vi "Get Entity Details.vi"(8 "error in (no error)":errorcluster, 10 "Entity Type":i32, 11 "Entity Table in":refnum<class "Entity Table.lvclass">) -> (0 "error out":errorcluster, 2 "Entity Details":cluster{"Name":string, "Status":string}[](array[cluster]), 3 "Entity Table out":refnum<class "Entity Table.lvclass">)   [LabVIEW 2020, in "Entity Table.lvclass"]
doc: "Copy out the details of one set of Entities. This is intended to aid in creating a status display."
uses:
  Entity Table.lvclass
  Entity Table.lvclass/Entity Table.ctl
  Entity Data.ctl
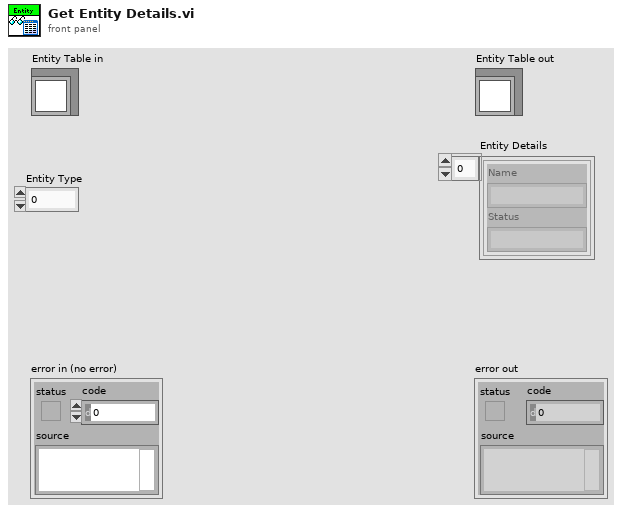
[diagram p1: front panel]
types:
  T1 = typedef "Entity Table.lvclass/Entity Data.ctl" = cluster{"Name":string, "Status":string}
  T2 = typedef "Entity Table.lvclass/Entity Table Element.ctl" = cluster{"Entity":refnum<class "Message Enqueuer.lvclass">[], "Entity Data":T1[]}
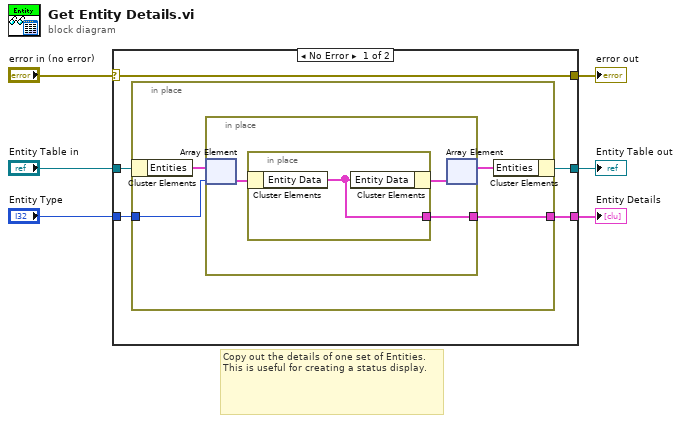
[diagram p0: block diagram]
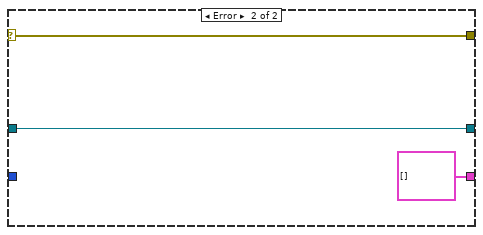
[diagram p2: hidden frame]
diagram:
  # "Copy out the details of one set of Entities.  This is useful for creating a status display."
  n1 = case shown="No Error" "error in (no error)" {
    selector: "error in (no error)" -> [w11 w22]
    tunnel: [w11 w22] -> w5
    tunnel: [w8 w21] -> w3
    tunnel: "Entity Table in" -> [w10 w21]
    tunnel: "Entity Type" -> [w9 _]
    tunnel: [w7 T1[] [] ("Entity Data")] -> w1
    frame No Error {
      n2 = in-place "In Place Element Structure" {
        in-place-border: w9 -> [w14]
        in-place-border: [w12] -> w7
        n3 = in-place-cluster #1 ("Unbundle / Bundle Elements")(w10) -> ("Entities"=w15:T2[])
        n4 = in-place "In Place Element Structure" {
          in-place-border: [w16] -> w12
          n5 = in-place-array #2 ("Array Index / Replace Elements")(w15, w14) -> (w18:T2)
          n6 = in-place "In Place Element Structure" {
            in-place-border: [w19] -> w16
            n7 = in-place-cluster #3 ("Unbundle / Bundle Elements")(w18) -> ("Entity Data"=w19:T1[])
            n8 = in-place-cluster #3 ("Unbundle / Bundle Elements")("Entity Data"=w19) -> (w17:T2)
          }
          n9 = in-place-array #2 ("Array Index / Replace Elements")(w17) -> (w13:T2[])  [unwired: 1 out]
        }
        n10 = in-place-cluster #1 ("Unbundle / Bundle Elements")("Entities"=w13) -> (w8:refnum<class "Entity Table.lvclass">)
      }
    }
    frame Error {
    }
  }
  "error out" <- w5
  "Entity Table out" <- w3
  "Entity Details" <- w1
